vi "Launcher.vi"() -> ()   [LabVIEW 2020, in "HIJ Vision App IMAQdx Display.lvlib"]
uses:
  HIJ Vision App IMAQdx Display.lvlib
  <vilib>/userdefined/High Color/IMAQdx.ctl
  HIJ Vision App IMAQdx Display/HIJ Vision App IMAQdx Display.lvclass
  C:/Users/AlexK/work/LabVIEW Programme/HIJ-Vision-Example-Project/Submodules/HIJ-Vision/Application Base Actors/HIJ Vision Camera App/HIJ Vision Camera App/HIJ Vision Camera App.lvclass
  C:/Users/AlexK/work/LabVIEW Programme/HIJ-Vision-Example-Project/Submodules/HIJ-Vision/Application Base Actors/HIJ Vision Application/HIJ Vision Application/HIJ Vision Application.lvclass
  C:/Program Files (x86)/National Instruments/LabVIEW 2020/vi.lib/ActorFramework/Actor/Actor.lvclass
  Display Actors/HIJ IMAQdx Display/AF IMAQ Display/HIJ IMAQdx Display.lvclass
  C:/Users/AlexK/work/LabVIEW Programme/HIJ-Vision-Example-Project/Submodules/HIJ-Vision/Display Actors/HIJ Vision Display/HIJ Vision Display/HIJ Vision Display.lvclass
  Display Actors/HIJ Vision Display/HIJ Vision Display/HIJ Vision Display.lvclass/HIJ Vision Display.ctl
  Display Actors/HIJ IMAQdx Display/AF IMAQ Display/HIJ IMAQdx Display.lvclass/HIJ IMAQdx Display.ctl
  Display Actors/HIJ Vision Display/HIJ Vision Display/Write WorkDir.vi
  Display Actors/HIJ IMAQdx Display/AF IMAQ Display/Write ConfigDir.vi
  <vilib>/Utility/config.llb/Read Key (Path).vi
  <vilib>/Utility/config.llb/Read Key (String).vi
  Application Base Actors/HIJ Vision Camera App/HIJ Vision Camera App/Write Camera Name.vi
  Application Base Actors/HIJ Vision Camera App/HIJ Vision Camera App/Write Start Acquisition.vi
  Application Base Actors/HIJ Vision Application/HIJ Vision Application/Write HIJ Vision Display.vi
  <vilib>/Utility/config.llb/Write Key (Path).vi
  <vilib>/Utility/config.llb/Write Key (String).vi
  <vilib>/ActorFramework/Actor/Actor.lvclass
  <vilib>/Utility/config.llb/NI_LVConfig.lvlib
panel:
  in  "UI Cnfg":path
  in  "CLine Parameter":string
  in  "RUN_STOP":bool=TRUE
  in  "Start WorkDir":path=path "C:/Users/user/Desktop/test/WorkDir"
  in  "Start ConfigDir":path=path "C:/Users/user/Desktop/test/ConfigDir"
  in  "Start Camera":T1="TestCam"
  out "error out":errorcluster
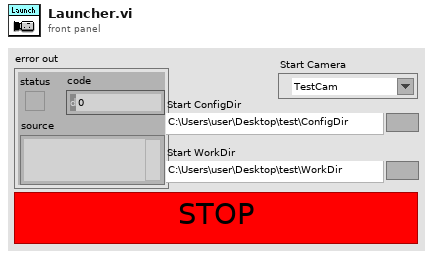
[diagram p1: front panel]
types:
  T1 = typedef "IMAQdx.ctl" = refnum<k21>
  T2 = typedef "NI_LVConfig.lvlib/Config Data RefNum.ctl" = refnum<k1>
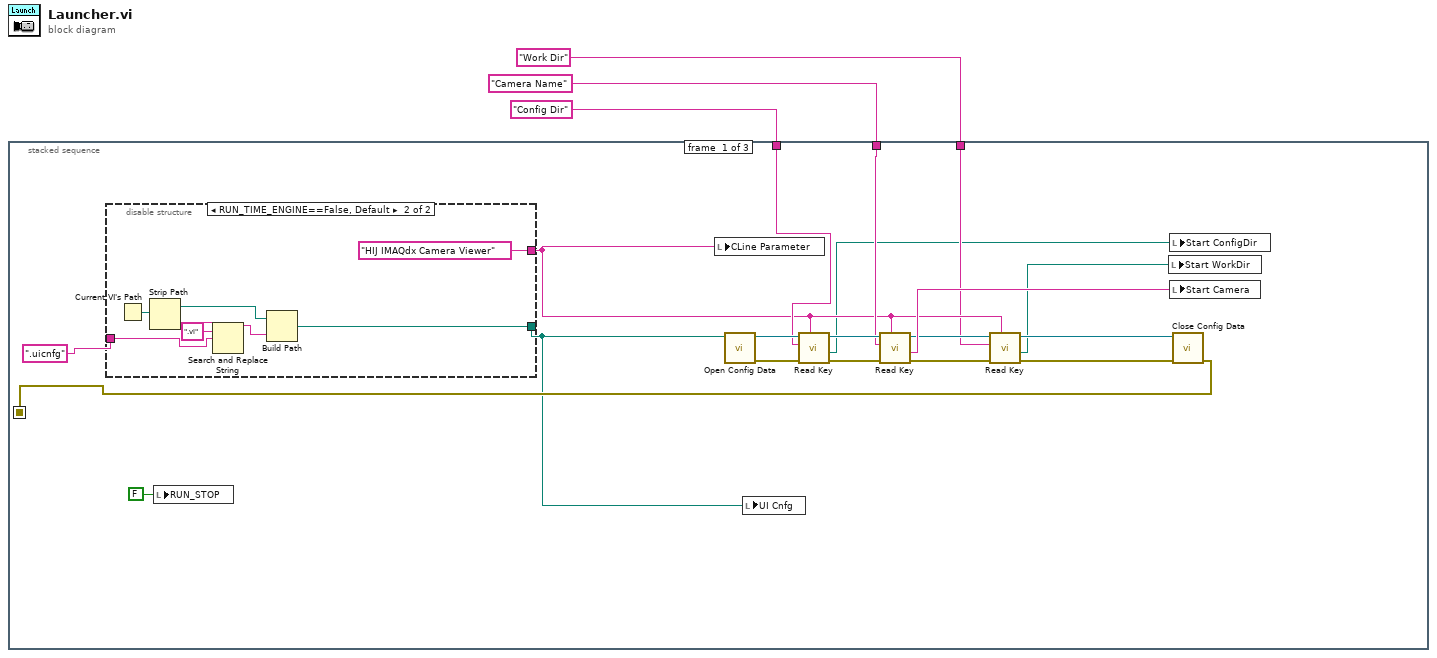
[diagram p0: block diagram]
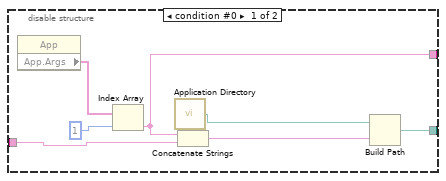
[diagram p2: hidden frame]
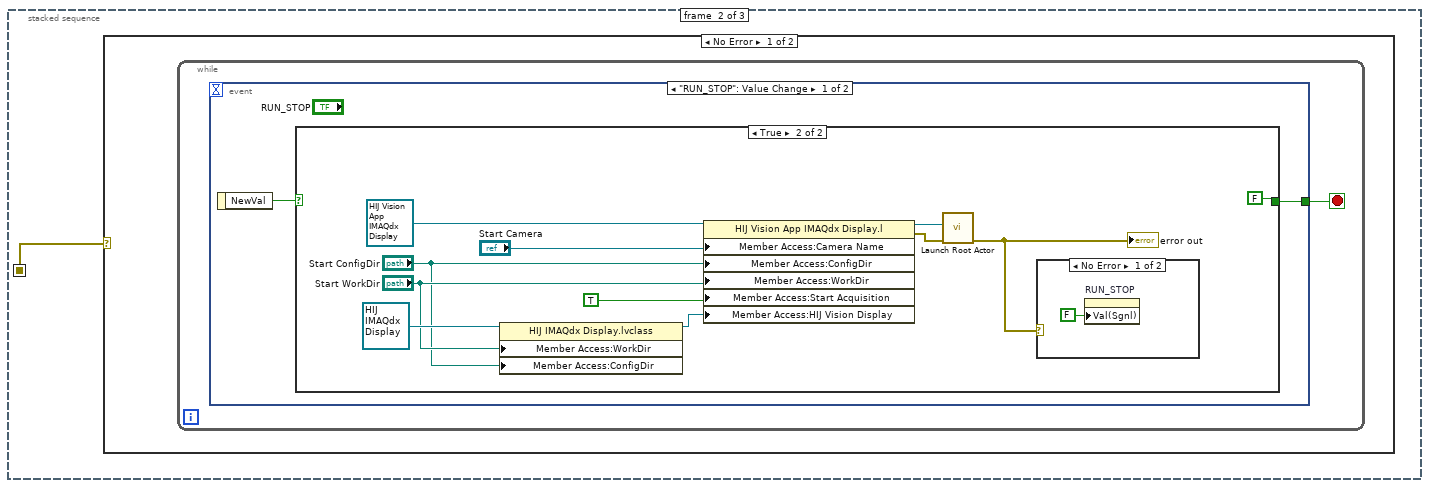
[diagram p3: hidden frame]
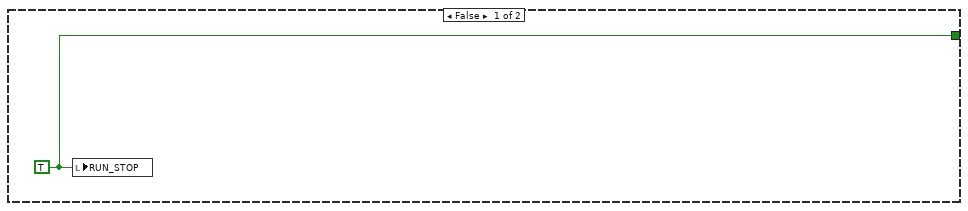
[diagram p4: hidden frame]
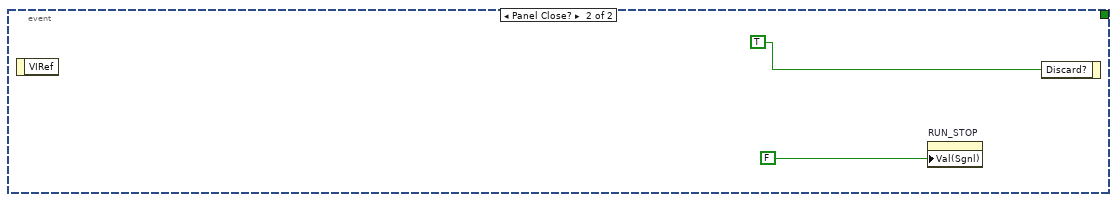
[diagram p6: hidden frame]
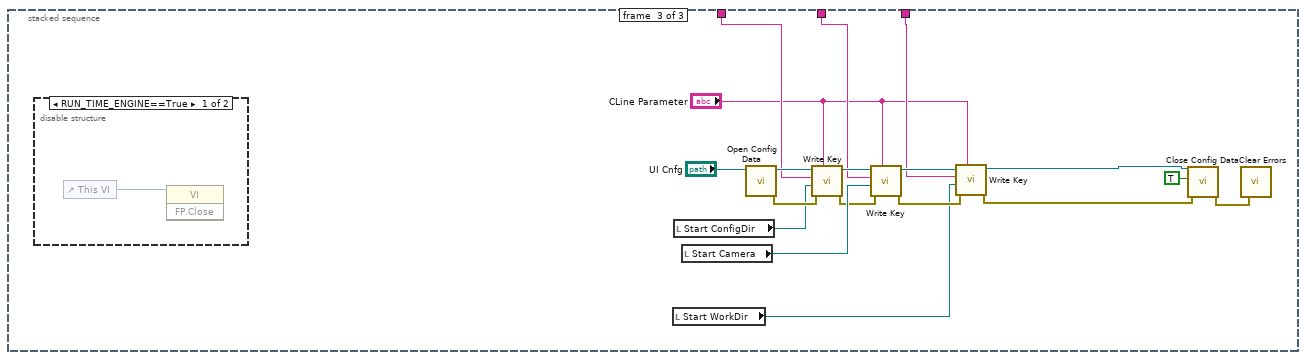
[diagram p8: hidden frame]
diagram:
  n1 = stacked-sequence {
    seq-local: [w15 _ _] -> [_ w38 _]
    tunnel: "Camera Name" ("key") -> [w17 _ w70]
    tunnel: "Config Dir" ("key") -> [w16 _ w71]
    tunnel: "Work Dir" ("key") -> [w6 _ w58]
    frame #0 {
      n2 = disable-structure shown="RUN_TIME_ENGINE==False, Default" {
        disable-tunnel: [w25 w31] -> w13
        disable-tunnel: ".uicnfg" ("string") -> [w24 w34]
        disable-tunnel: [w23 "HIJ IMAQdx Camera Viewer"] -> w7
        frame condition #0 {
          n3 = property class="App"() -> ("App.Args"=w29:string[])  [unwired: 2 in, 2 out]
          n4 = Index Array(array=w29, index=1) -> (element=w23:string)
          n5 = call <vilib>:"Application Directory.vi"() -> ("Application Directory"=w27:path)
          n6 = Concatenate Strings(w23, w24) -> (w26:string)
          n7 = Build Path(base path=w27, name or relative path=w26) -> (appended path=w25:path)
        }
        frame condition #1 (active) {
          n8 = Current VI's Path() -> (path=w37:path)
          n9 = Strip Path(path=w37) -> (stripped path=w32:path, name=w36:string)
          n10 = Search and Replace String(input string=w36, search string=".vi", replace string=w34) -> (result string=w33:string)  [unwired: 5 in, 3 out]
          n11 = Build Path(base path=w32, name or relative path=w33) -> (appended path=w31:path)
        }
      }
      n12 = local write "RUN_STOP"(FALSE ("RUN_STOP")) -> ()
      n13 = local write "CLine Parameter"(w7) -> ()
      n14 = call <vilib>:"Open Config Data.vi"("configuration file path"=w13) -> ("error out"=w19:errorcluster, "refnum"=w18:T2)  [unwired: 8 in, 1 out]
      n15 = local write "UI Cnfg"(w13) -> ()
      n16 = call-poly <vilib>:"Read Key.vi"("section"=w7, "error in (no error)"=w19, "key"=w16, "refnum"=w18) -> ("error out"=w20:errorcluster, "value"=w4:path, "refnum out"=w21:T2)  [unwired: 4 in, 1 out]
      n17 = call-poly <vilib>:"Read Key.vi"("section"=w7, "error in (no error)"=w20, "key"=w17, "refnum"=w21) -> ("error out"=w11:errorcluster, "value"=w12:string, "refnum out"=w9:T2)  [unwired: 4 in, 1 out]
      n18 = call-poly <vilib>:"Read Key.vi"("section"=w7, "error in (no error)"=w11, "key"=w6, "refnum"=w9) -> ("error out"=w10:errorcluster, "value"=w5:path, "refnum out"=w8:T2)  [unwired: 4 in, 1 out]
      n19 = local write "Start WorkDir"(w5) -> ()
      n20 = local write "Start ConfigDir"(w4) -> ()
      n21 = local write "Start Camera"(w12) -> ()
      n22 = call <vilib>:"Close Config Data.vi"("error in (no error)"=w10, "refnum"=w8) -> ("error out"=w15:errorcluster)  [unwired: 8 in, 1 out]
    }
    frame #1 {
      n23 = case shown="No Error" w38 {
        frame No Error {
          n24 = while {
            stop <- w39 stop-if-true
            n25 = event shown="[0] \"RUN_STOP\": Value Change" {
              selector: _ -> [_ _]
              dyn-events: _ -> [_ _]
              timeout: _ -> [_ _]
              tunnel: [w41 _] -> w39
              event "RUN_STOP": Value Change {
                n26 = event-data() -> ("NewVal"=w40:bool)  [unwired: 1 in]
                n27 = case shown="True" w40 {
                  tunnel: [w42 FALSE] -> w41
                  frame False {
                    w42 = TRUE ("RUN_STOP")
                    n28 = local write "RUN_STOP"(w42) -> ()
                  }
                  frame True {
                    n29 = property class="HIJ IMAQdx Display.lvclass"(reference=refnum<class "HIJ IMAQdx Display.lvclass"> refnum ("HIJ IMAQdx Display.lvlib:HIJ IMAQdx Display.lvclass"), "Member Access:WorkDir"="Start WorkDir", "Member Access:ConfigDir"="Start ConfigDir") -> (reference out=w45:refnum<class "HIJ IMAQdx Display.lvclass">)  [unwired: 1 in, 1 out]
                    n30 = property class="HIJ Vision App IMAQdx Display.l"(reference=refnum<class "HIJ Vision App IMAQdx Display.lvclass"> refnum ("Launch IMAQ Display.lvlib:Launch IMAQ Display.lvclass"), "Member Access:Camera Name"="Start Camera", "Member Access:ConfigDir"="Start ConfigDir", "Member Access:WorkDir"="Start WorkDir", "Member Access:Start Acquisition"=TRUE ("Start Acquisition"), "Member Access:HIJ Vision Display"=w45) -> (reference out=w49:refnum<class "HIJ Vision App IMAQdx Display.lvclass">, error out=w50:errorcluster)  [unwired: 1 in]
                    n31 = call <vilib>:"Launch Root Actor.vi"("error in (no error)"=w50, "Actor"=w49) -> ("error out"=w47:errorcluster)  [unwired: 8 in, 1 out]
                    "error out" <- w47
                    n32 = case shown="No Error" w47 {
                      frame No Error {
                        n33 = property on="RUN_STOP" class="Bool (strict)"("Val(Sgnl)"=FALSE ("Value (Signaling)")) -> ()  [unwired: 2 in, 2 out]
                      }
                      frame Error {
                      }
                    }
                  }
                }
              }
              event Panel Close? {
                n34 = event-data() -> ()  [unwired: 1 in, 1 out]
                n35 = property on="RUN_STOP" class="Bool (strict)"("Val(Sgnl)"=FALSE ("Value (Signaling)")) -> ()  [unwired: 2 in, 2 out]
                n36 = event-data("Discard?"=TRUE) -> ()  [unwired: 1 in, 1 out]
              }
            }
          }
        }
        frame Error {
        }
      }
    }
    frame #2 {
      n37 = disable-structure shown="RUN_TIME_ENGINE==True" {
        frame condition #0 {
          n38 = control-ref of="This VI"() -> (w75:refnum<vi>)
          n39 = invoke class="VI" method="FP.Close"(reference=w75) -> ()  [unwired: 2 in, 3 out]
        }
        frame condition #1 (active) {
        }
      }
      n40 = local read "Start WorkDir"() -> (w59:path)
      n41 = local read "Start ConfigDir"() -> (w64:path)
      n42 = local read "Start Camera"() -> (w69:T1)
      n43 = call <vilib>:"Open Config Data.vi"("configuration file path"="UI Cnfg") -> ("error out"=w68:errorcluster, "refnum"=w73:T2)  [unwired: 8 in, 1 out]
      n44 = call-poly <vilib>:"Write Key.vi"("section"="CLine Parameter", "error in (no error)"=w68, "value"=w64, "key"=w71, "refnum"=w73) -> ("error out"=w67:errorcluster, "refnum out"=w74:T2)  [unwired: 4 in, 1 out]
      n45 = call-poly <vilib>:"Write Key.vi"("section"="CLine Parameter", "error in (no error)"=w67, "value"=w69, "key"=w70, "refnum"=w74) -> ("error out"=w62:errorcluster, "refnum out"=w63:T2)  [unwired: 4 in, 1 out]
      n46 = call-poly <vilib>:"Write Key.vi"("section"="CLine Parameter", "error in (no error)"=w62, "value"=w59, "key"=w58, "refnum"=w63) -> ("error out"=w61:errorcluster, "refnum out"=w60:T2)  [unwired: 4 in, 1 out]
      n47 = call <vilib>:"Close Config Data.vi"("error in (no error)"=w61, "write file if changed (T)"=TRUE, "refnum"=w60) -> ("error out"=w66:errorcluster)  [unwired: 7 in, 1 out]
      n48 = call <vilib>:"Clear Errors.vi"("error in (no error)"=w66) -> ()  [unwired: 5 in, 2 out]
    }
  }
